vi "Varient_number_check.vi"(8 "error in":errorcluster, 10 "Varient path":path, 11 "Varient No.":u16) -> (0 "error out":errorcluster, 1 "Batch Size":i32, 2 "Varient Number":i32, 3 "Part Name":string, 4 "PART_NO":string, 5 "TORISHI_CODE":string)   [LabVIEW 2017]
uses:
  <vilib>/Utility/config.llb/Read Key (I32).vi
  <vilib>/Utility/config.llb/Read Key (String).vi
  <vilib>/Utility/config.llb/NI_LVConfig.lvlib
panel:
  # "Varient no. check"
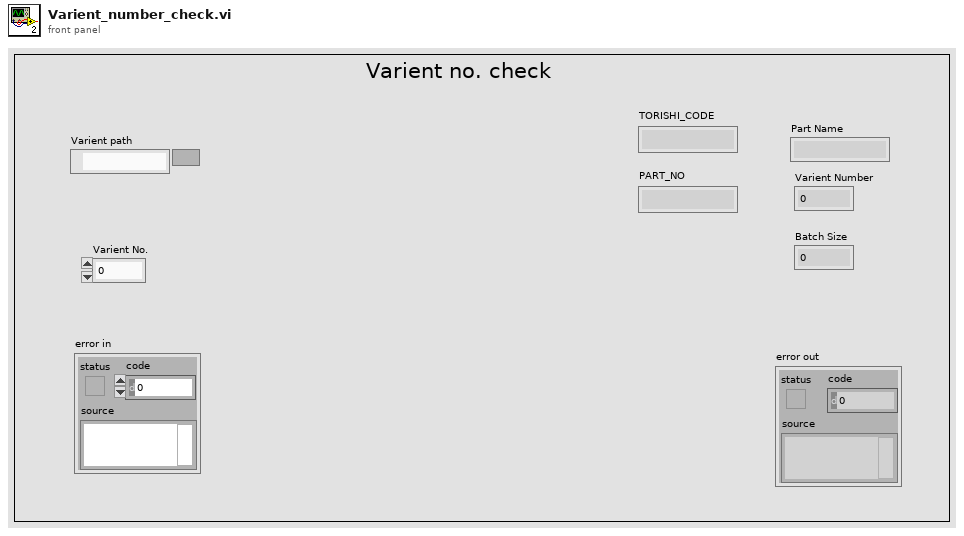
[diagram p1: front panel]
types:
  T1 = typedef "NI_LVConfig.lvlib/Config Data RefNum.ctl" = refnum<k1>
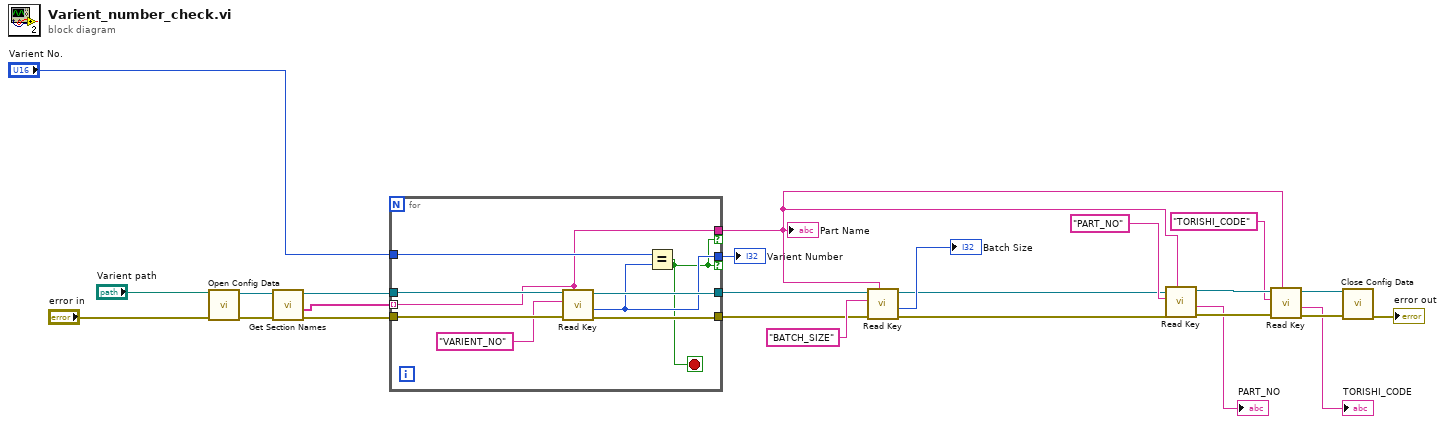
[diagram p0: block diagram]
diagram:
  n1 = call <vilib>:"Open Config Data.vi"("error in (no error)"="error in", "configuration file path"="Varient path") -> ("error out"=w24:errorcluster, "refnum"=w25:T1)  [unwired: 7 in, 1 out]
  n2 = call <vilib>:"Get Section Names.vi"("error in (no error)"=w24, "refnum"=w25) -> ("error out"=w22:errorcluster, "section names"=w20:string[], "refnum out"=w21:T1)  [unwired: 7 in]
  n3 = for {
    tunnel: w20 -> [w27] mode=indexing
    tunnel: w21 -> [w32]
    tunnel: [w31] -> w15
    tunnel: w22 -> [w34]
    tunnel: [w33] -> w16
    tunnel: [w28] -> w18 if=w26
    tunnel: "Varient No." -> [w29]
    tunnel: [w27] -> w5 if=w26
    stop <- w26 stop-if-true
    n4 = call-poly <vilib>:"Read Key.vi"("section"=w27, "error in (no error)"=w34, "key"="VARIENT_NO" ("name or relative path"), "refnum"=w32) -> ("error out"=w33:errorcluster, "value"=w28:i32, "refnum out"=w31:T1)  [unwired: 4 in, 1 out]
    n5 = Equal?(x=w29, y=w28) -> (x = y?=w26:bool)
  }
  "Varient Number" <- w18
  "Part Name" <- w5
  n6 = call-poly <vilib>:"Read Key.vi"("section"=w5, "error in (no error)"=w16, "key"="BATCH_SIZE" ("name or relative path"), "refnum"=w15) -> ("error out"=w7:errorcluster, "value"=→"Batch Size":i32, "refnum out"=w9:T1)  [unwired: 4 in, 1 out]
  n7 = call-poly <vilib>:"Read Key.vi"("section"=w5, "error in (no error)"=w7, "key"="PART_NO", "refnum"=w9) -> ("error out"=w12:errorcluster, "value"=→"PART_NO":string, "refnum out"=w13:T1)  [unwired: 4 in, 1 out]
  n8 = call-poly <vilib>:"Read Key.vi"("section"=w5, "error in (no error)"=w12, "key"="TORISHI_CODE", "refnum"=w13) -> ("error out"=w6:errorcluster, "value"=→"TORISHI_CODE":string, "refnum out"=w8:T1)  [unwired: 4 in, 1 out]
  n9 = call <vilib>:"Close Config Data.vi"("error in (no error)"=w6, "refnum"=w8) -> ("error out"=→"error out":errorcluster)  [unwired: 8 in, 1 out]
